vi "Get Owning Custom Device Ref.vi"(8 "error in":errorcluster, 11 "Item Ref":T1 format="%.0x") -> (0 "error out":errorcluster, 3 "Custom Device Ref":T1 format="%.0x")   [LabVIEW 2020, in "Communication Bus Template System Explorer.lvlib" / "Implementation.lvlib" / "System Explorer Dispatcher.lvclass"]
uses:
  System Explorer Dispatcher.lvclass
  NationalInstruments.VeriStand.SystemDefinitionAPI
  Scripting/Constants.vi
  Scripting/Communication Bus Template Scripting.lvlib
  <vilib>/NI VeriStand/Custom Device API/Custom Device Item Ref.ctl
  <vilib>/NI VeriStand/Custom Device API/Custom Device API.lvlib
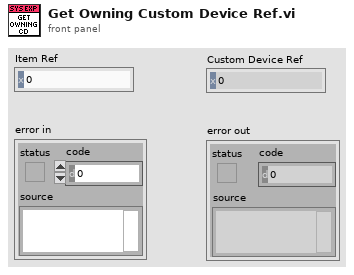
[diagram p1: front panel]
types:
  T1 = typedef "Custom Device API.lvlib/Custom Device Item Ref.ctl" = u64
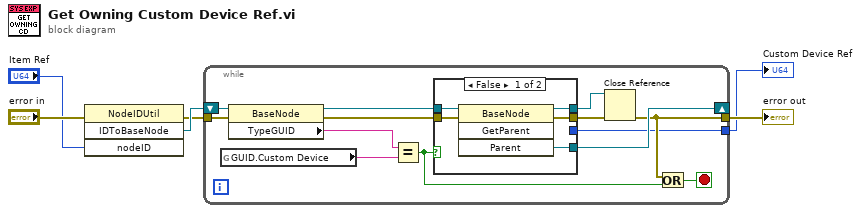
[diagram p0: block diagram]
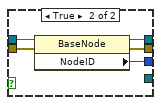
[diagram p2: hidden frame]
diagram:
  n1 = invoke class="NodeIDUtil" method="IDToBaseNode"(error in="error in", "nodeID"="Item Ref") -> (error out=w3:errorcluster, "IDToBaseNode"=w4:refnum<k24>)  [unwired: 2 in, 2 out]
  n2 = while {
    tunnel: w3 -> [w16]
    tunnel: [w8] -> w2
    shift-right: [w13] -> _
    shift-left: w4 -> [w19]
    tunnel: [w7] -> w1
    stop <- w15 stop-if-true
    n3 = global read "Constants.vi" "GUID.Custom Device"() -> (w17:string)
    n4 = property class="BaseNode"(reference=w19, error in=w16) -> (reference out=w14:refnum<k24>, error out=w12:errorcluster, "TypeGUID"=w18:string)
    n5 = Equal?(x=w18, y=w17) -> (x = y?=w9:bool)
    n6 = case shown="False" w9 {
      tunnel: w14 -> [w24 w27]
      tunnel: [w23 _] -> w13
      tunnel: w12 -> [w22 w28]
      tunnel: [w21 w26] -> w11
      tunnel: [w20 w29] -> w10
      tunnel: [_ w25] -> w7
      frame False {
        n7 = invoke class="BaseNode" method="GetParent"(reference=w24, error in=w22) -> (reference out=w20:refnum<k24>, error out=w21:errorcluster, "Parent"=w23:refnum<k24>)  [unwired: 2 in, 1 out]
      }
      frame True {
        n8 = property class="BaseNode"(reference=w27, error in=w28) -> (reference out=w29:refnum<k24>, error out=w26:errorcluster, "NodeID"=w25:u64)
      }
    }
    n9 = Close Reference(reference=w10, error in (no error)=w11) -> (error out=w8:errorcluster)
    n10 = Or(x=w8, y=w9) -> (x .or. y?=w15:bool)
  }
  "Custom Device Ref" <- w1
  "error out" <- w2
